vi "DAQmx Fill In Error Info.vi"(1 "depth":i32=1, 5 "status code":i32, 7 "extended error info":string, 11 "error in":errorcluster) -> (15 "error out":errorcluster)   [LabVIEW 2013]
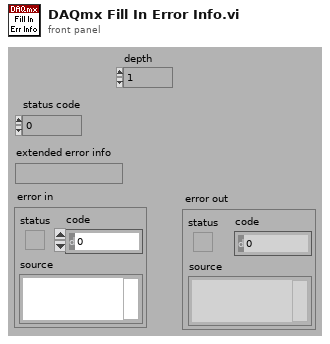
[diagram p1: front panel]
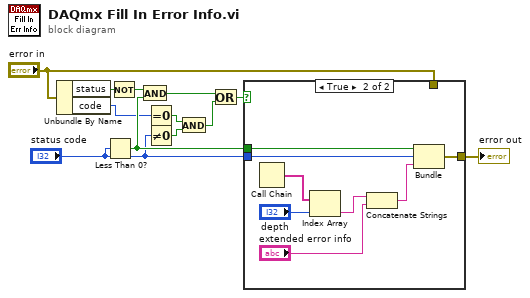
[diagram p0: block diagram]
diagram:
  n1 = Unbundle By Name("error in") -> ("status"=w4:bool, "code"=w9:i32)
  n2 = Less Than 0?(x="status code") -> (x < 0?=w10:bool)
  n3 = Not(x=w4) -> (.not. x?=w8:bool)
  n4 = And(x=w8, y=w10) -> (x .and. y?=w5:bool)
  n5 = Equal To 0?(x=w9) -> (x = 0?=w3:bool)
  n6 = Not Equal To 0?(x="status code") -> (x != 0?=w6:bool)
  n7 = And(x=w3, y=w6) -> (x .and. y?=w2:bool)
  n8 = Or(x=w5, y=w2) -> (x .or. y?=w1:bool)
  n9 = case shown="True" w1 {
    tunnel: [w13 w20] -> w11
    tunnel: "status code" -> [_ w19]
    tunnel: w10 -> [_ w18]
    tunnel: "error in" -> [w13 _]
    frame False {
    }
    frame True {
      n10 = Call Chain() -> (call chain=w16:string[])
      n11 = Index Array(array=w16, index="depth") -> (element=w14:string)
      n12 = Concatenate Strings(w14, "extended error info") -> (w21:string)
      n13 = Bundle(w18, "status code"=w19, w21) -> (w20:cluster{bool, "status code":i32, string})  [unwired: 1 out]
    }
  }
  "error out" <- w11
